vi "Start WiFi Hotspot.vi"(10 "Password":string, 11 "SSID":string) -> (0 "error out":errorcluster)   [LabVIEW 2015]
panel:
  out "return code":i32[](array[numeric])
  out "std error":string[](array[string])
  out "std output":string[](array[string])
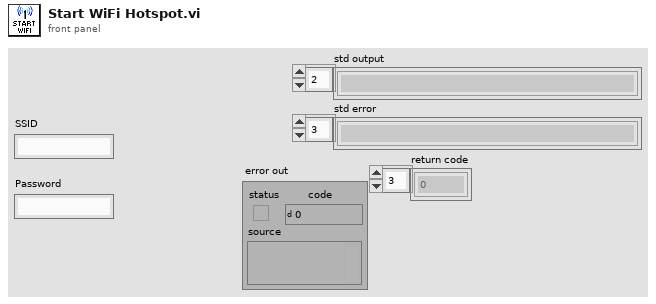
[diagram p1: front panel]
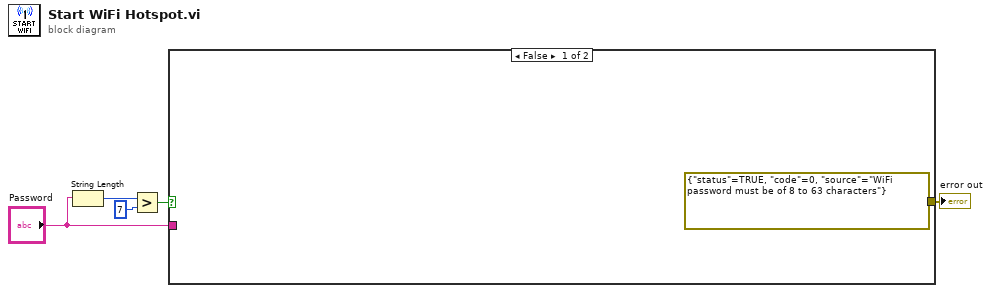
[diagram p0: block diagram]
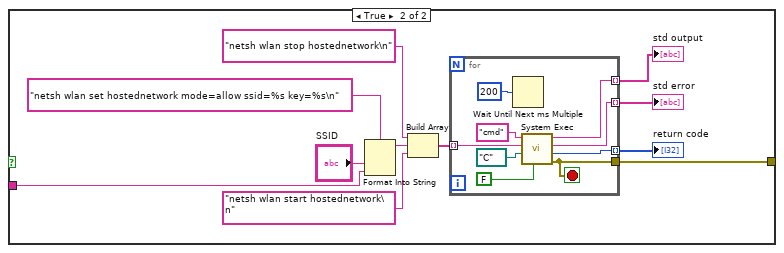
[diagram p2: hidden frame]
diagram:
  n1 = String Length(string="Password") -> (length=w4:i32)
  n2 = Greater?(x=w4, y=7) -> (0:w1:bool)
  n3 = case shown="False" w1 {
    tunnel: "Password" -> [_ w8]
    tunnel: [errorcluster {"status"=TRUE, "code"=0, "source"="WiFi password must be of 8 to 63 characters"} ("error out") w7] -> w2
    frame False {
    }
    frame True {
      n4 = Format Into String(format string="netsh wlan set hostednetwork mode=allow ssid=%s key=%s\n", "SSID", w8) -> (resulting string=w14:string)  [unwired: 2 in, 1 out]
      n5 = Build Array("netsh wlan stop hostednetwork\n" ("format string"), w14, "netsh wlan start hostednetwork\n" ("format string")) -> (w12:string[])
      n6 = for {
        tunnel: w12 -> [w25] mode=indexing
        tunnel: [w26] -> w7
        tunnel: [w20] -> w11 mode=indexing
        tunnel: [w19] -> w10 mode=indexing
        tunnel: [w18] -> w9 mode=indexing
        stop <- w26 stop-if-true
        n7 = Wait Until Next ms Multiple(millisecond multiple=u32 200) -> ()  [unwired: 1 out]
        n8 = call <vilib>:"System Exec.vi"("run minimized? (F)"=FALSE, "working directory"=path "C:/", "standard input"=w25, "command line"="cmd") -> ("error out"=w26:errorcluster, "return code"=w18:i32, "standard error"=w19:string, "standard output"=w20:string)  [unwired: 4 in]
      }
      "std output" <- w11
      "std error" <- w10
      "return code" <- w9
    }
  }
  "error out" <- w2
